vi "laser_set_point.vi"() -> ()   [LabVIEW 2011]
uses:
  <vilib>/DAQmx/write.llb/DAQmx Write (Analog DBL 1Chan 1Samp).vi
  PS_Global.vi
  <vilib>/DAQmx/create/channels.llb/DAQmx Create Channel (AO-Voltage-Basic).vi
  <vilib>/DAQmx/miscellaneous.llb/DAQmx Fill In Error Info.vi
panel:
  in  "Voltage Set":dbl
  in  "Maximum Value 2":dbl=10.0 caption="Maximum Value" format="%0.2f"
  in  "Minimum Value 2":dbl=-10.0 caption="Minimum Value" format="%0.2f"
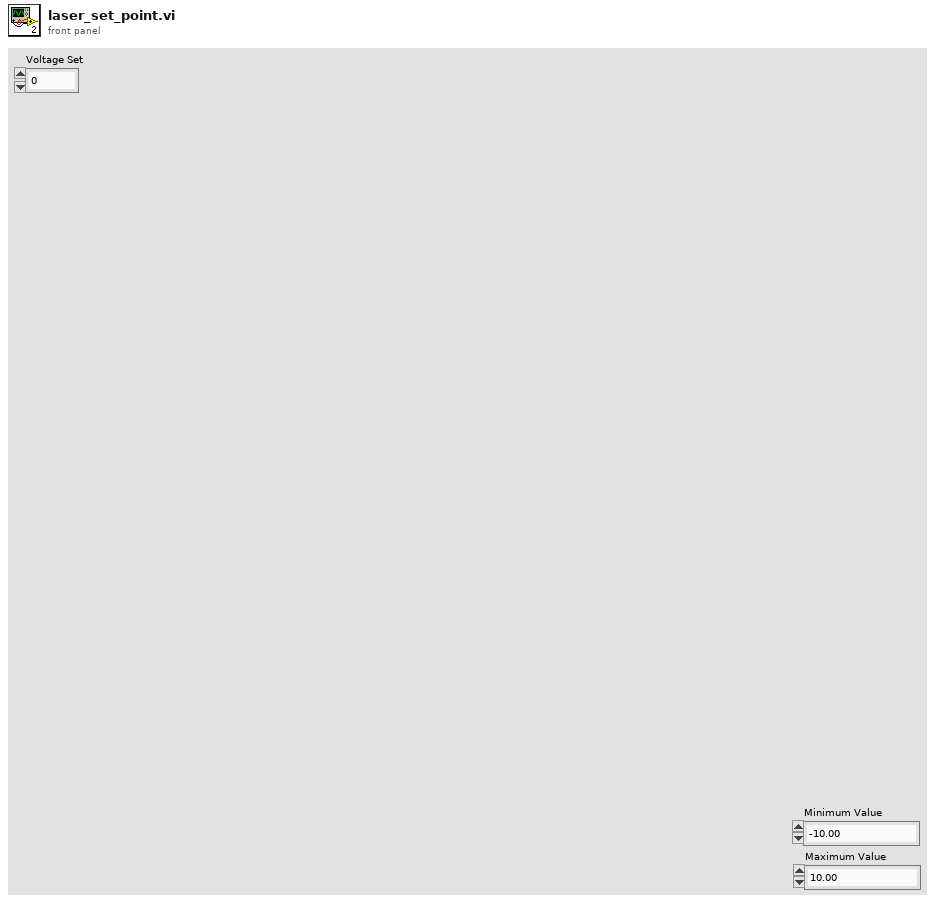
[diagram p1: front panel]
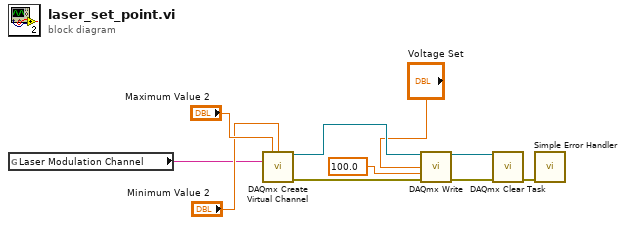
[diagram p0: block diagram]
diagram:
  n1 = global read "PS_Global.vi" "Laser Modulation Channel"() -> (w1:tag)
  n2 = call-poly <vilib>:"DAQmx Create Virtual Channel.vi"("maximum value"="Maximum Value 2", "minimum value"="Minimum Value 2", "physical channels"=w1) -> ("task out"=w6:refnum<k21>, "error out"=w5:errorcluster)  [unwired: 11 in]
  n3 = call-poly <vilib>:"DAQmx Write.vi"("task/channels in"=w6, "data"="Voltage Set", "timeout"=100.0, "error in"=w5) -> ("task out"=w9:refnum<k21>, "error out"=w8:errorcluster)  [unwired: 9 in, 1 out]
  n4 = call <vilib>:"DAQmx Clear Task.vi"("task in"=w9, "error in"=w8) -> ("error out"=w10:errorcluster)  [unwired: 13 in]
  n5 = call <vilib>:"Simple Error Handler.vi"("error in (no error)"=w10) -> ()  [unwired: 4 in, 5 out]
